vi "S2C_ParseSettings.vi"(8 "Error In":errorcluster, 11 "Table Data":string[](array[string])) -> (0 "Error Out":errorcluster, 3 "Result":string)   [LabVIEW 2015]
doc: "If enabled, saves the test report to the local drive."
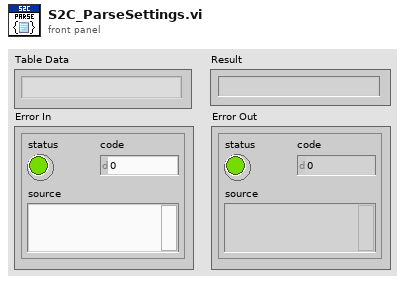
[diagram p1: front panel]
types:
  T1 = cluster{"Step Type":string, "High Limit":string, "High Limit Comparison":string, "Low Limit":string, "Low Limit Comparison":string, "Units":string}
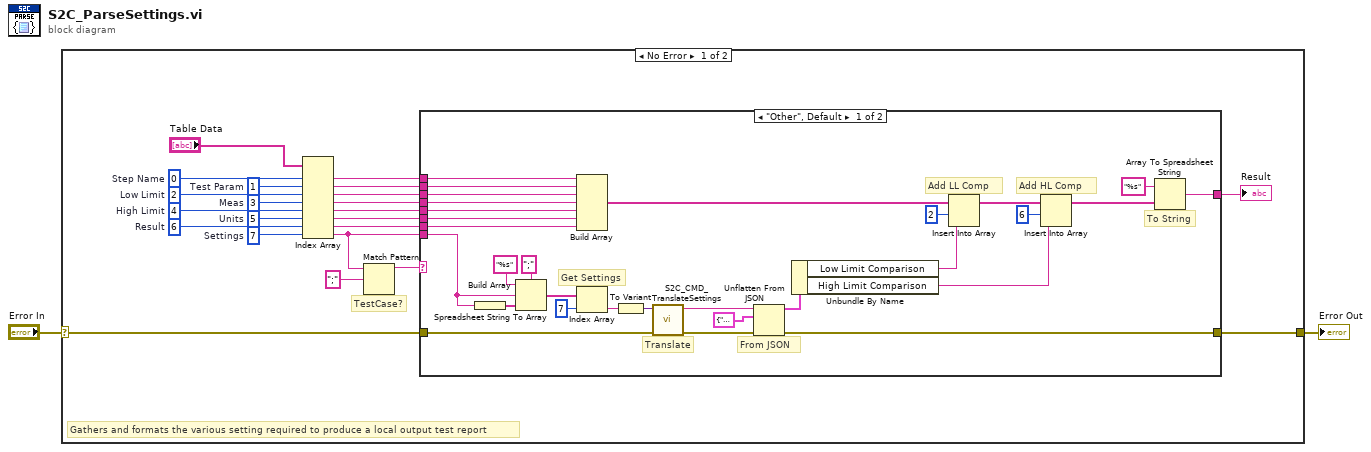
[diagram p0: block diagram]
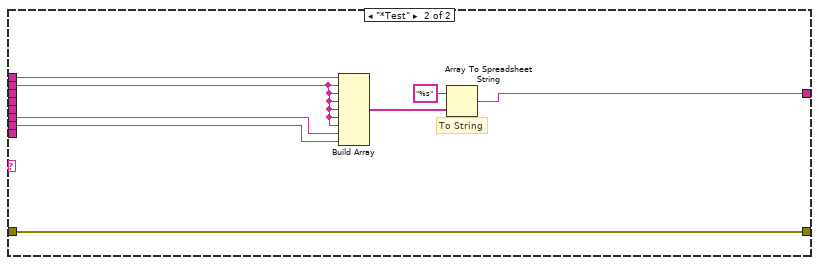
[diagram p2: hidden frame]
diagram:
  n1 = case shown="No Error" "Error In" {
    selector: "Error In" -> [w24 w63]
    tunnel: [w23 w63] -> w1
    frame No Error {
      w15 = 7  # Settings
      w16 = 6  # Result
      w17 = 5  # Units
      w18 = 4  # High Limit
      w19 = 3  # Meas
      w20 = 2  # Low Limit
      w21 = 1  # Test Param
      w22 = 0  # Step Name
      # "TestCase?"
      # "Gathers and formats the various setting required to produce a local output test report"
      n2 = Index Array(array="Table Data", index #1=w22, index #2=w21, index #3=w20, index #4=w19, index #5=w18, index #6=w17, index #7=w16, index #8=w15) -> (element #1=w13:string, element #2=w12:string, element #3=w11:string, element #4=w10:string, element #5=w9:string, element #6=w8:string, element #7=w7:string, element #8=w5:string)
      n3 = Match Pattern(string=w5, regular expression=";") -> (before substring=w3:string)  [unwired: 1 in, 3 out]
      n4 = case shown="\"Other\", Default" w3 {
        tunnel: w24 -> [w54 w59]
        tunnel: [w53 w59] -> w23
        tunnel: w13 -> [w46 w61]
        tunnel: w12 -> [w45 w57]
        tunnel: w11 -> [w44 _]
        tunnel: w10 -> [w43 _]
        tunnel: w9 -> [w42 _]
        tunnel: w8 -> [w41 w56]
        tunnel: w7 -> [w40 w55]
        tunnel: [w26 w60] -> w6
        tunnel: w5 -> [w25 _]
        frame "Other", Default {
          # "To String"
          # "Add HL Comp"
          # "Add LL Comp"
          # "From JSON"
          # "Translate"
          # "Get Settings"
          n5 = Build Array(w25) -> (w30:string[])
          n6 = Spreadsheet String To Array(delimiter (Tab)=";", format string="%s", spreadsheet string=w25, array type (2D Dbl)=w30) -> (array=w33:string[])
          n7 = Build Array(w46, w45, w44, w43, w42, w41, w40) -> (w39:string[])
          n8 = Index Array(array=w33, index=7) -> (element=w29:string)
          n9 = To Variant(anything=w29) -> (Variant=w51:variant)
          n10 = call "S2C_CMD_TranslateSettings.vi"("Error In"=w54, "Data"=w51) -> ("Error Out"=w50:errorcluster, "JSON Cluster"=w48:string)  [unwired: 8 in]
          n11 = Unflatten From JSON(JSON string=w48, type and defaults=T1 {"Step Type"="", "High Limit"="", "High Limit Comparison"="", "Low Limit"="", "Low Limit Comparison"="", "Units"=""}, error in (no error)=w50) -> (value=w47:T1, error out=w53:errorcluster)  [unwired: 4 in]
          n12 = Unbundle By Name(w47) -> ("Low Limit Comparison"=w28:string, "High Limit Comparison"=w27:string)
          n13 = Insert Into Array(array=w39, index=2, new element=w28) -> (w36:string[])
          n14 = Insert Into Array(array=w36, index=6, new element=w27) -> (w35:string[])
          n15 = Array To Spreadsheet String(array=w35, 3:"%s" ("format string")) -> (spreadsheet string=w26:string)  [unwired: 1 in]
        }
        frame "*Test" {
          # "To String"
          n16 = Build Array(w61, w57, w57, w57, w57, w57, w57, w56, w55) -> (w58:string[])
          n17 = Array To Spreadsheet String(array=w58, 3:"%s" ("format string")) -> (spreadsheet string=w60:string)  [unwired: 1 in]
        }
      }
      "Result" <- w6
    }
    frame Error {
    }
  }
  "Error Out" <- w1
